vi "Util - Unbundle - 4Ch.vi"(8 "in3":T1, 9 "in2":T1, 10 "in1":T1, 11 "in0":T1) -> (2 "Timed Out?":bool, 3 "DSP Overflow":bool)   [LabVIEW 2015, in "DDC_7976R_v1.lvlib"]
uses:
  DDC_7976R_v1.lvlib
  Typedef - internal -02.ctl
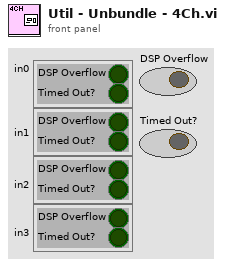
[diagram p1: front panel]
types:
  T1 = typedef "DDC_7976R_v1.lvlib/Typedef - internal -02.ctl" = cluster{"DSP Overflow":bool, "Timed Out?":bool}
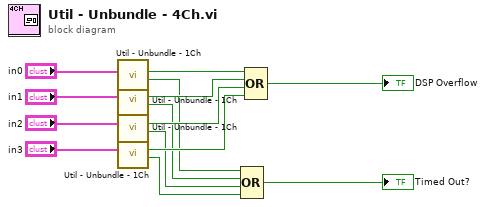
[diagram p0: block diagram]
diagram:
  n1 = call "Util - Unbundle - 1Ch.vi"("output"="in0") -> ("Timed Out?"=w3:bool, "DSP Overflow"=w10:bool)  [unwired: 9 in]
  n2 = call "Util - Unbundle - 1Ch.vi"("output"="in1") -> ("Timed Out?"=w4:bool, "DSP Overflow"=w9:bool)  [unwired: 9 in]
  n3 = call "Util - Unbundle - 1Ch.vi"("output"="in2") -> ("Timed Out?"=w5:bool, "DSP Overflow"=w8:bool)  [unwired: 9 in]
  n4 = call "Util - Unbundle - 1Ch.vi"("output"="in3") -> ("Timed Out?"=w6:bool, "DSP Overflow"=w7:bool)  [unwired: 9 in]
  n5 = Compound Arithmetic op=OR(w3, w4, w5, w6) -> (→"Timed Out?":bool)
  n6 = Compound Arithmetic op=OR(w10, w9, w8, w7) -> (→"DSP Overflow":bool)
